vi "(Depricated) Handle Sample In.vi"(8 "error in (no error)":errorcluster, 10 "Sample":refnum<class "Sample.lvclass">, 11 "Transfer Line in":refnum<class "Transfer Line.lvclass">=refnum) -> (0 "error out":errorcluster, 3 "Transfer Line out":refnum<class "Transfer Line.lvclass">)   [LabVIEW 2015]
uses:
  Transfer Line.lvclass
  subs/Sample/Sample.lvclass
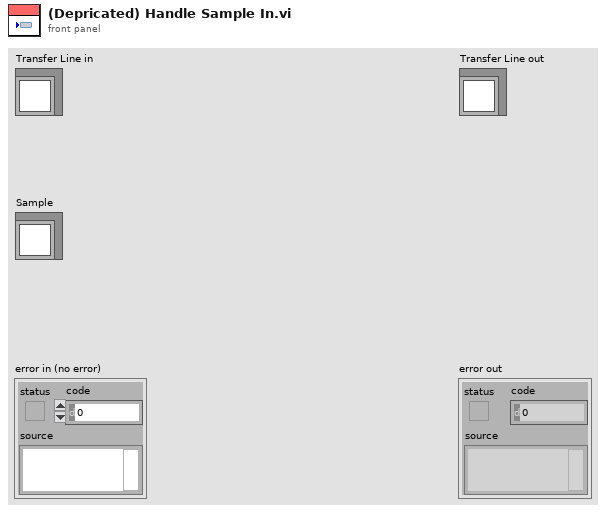
[diagram p1: front panel]
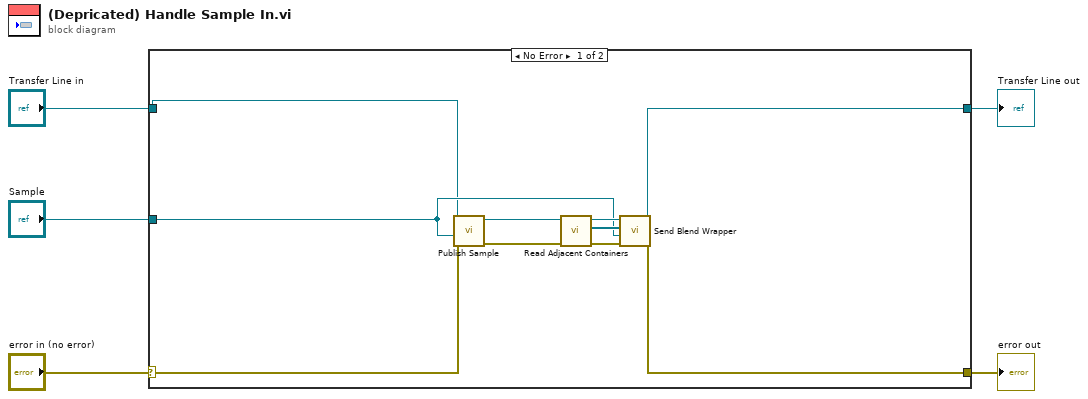
[diagram p0: block diagram]
diagram:
  n1 = case shown="No Error" "error in (no error)" {
    selector: "error in (no error)" -> [w8 w17]
    tunnel: [w11 w17] -> w3
    tunnel: [w10 w16] -> w4
    tunnel: "Transfer Line in" -> [w7 w16]
    tunnel: "Sample" -> [w9 _]
    frame No Error {
      n2 = call-dynamic "Publish Sample.vi"("error in (no error)"=w8, "Sample in"=w9, "Transfer Line in"=w7) -> ("error out"=w15:errorcluster, "Transfer Line out"=w6:refnum<class "Transfer Line.lvclass">)  [unwired: 7 in]
      n3 = call "Read Adjacent Containers.vi"("error in (no error)"=w15, "Transfer Line in"=w6) -> ("error out"=w14:errorcluster, "Adjacent Containers"=w12:refnum<class "Message Enqueuer.lvclass">[], "Transfer Line out"=w13:refnum<class "Transfer Line.lvclass">)  [unwired: 7 in]
      n4 = call-dynamic "Send Blend Wrapper.vi"("error in (no error)"=w14, "Sample to Blend"=w9, "Send to"=w12, "CO2 Actor in"=w13) -> ("error out"=w11:errorcluster, "CO2 Actor out"=w10:refnum<class "Transfer Line.lvclass">)  [unwired: 6 in]
    }
    frame Error {
    }
  }
  "error out" <- w3
  "Transfer Line out" <- w4
